vi "test_pid_1.vi"() -> ()   [LabVIEW 2018]
panel:
  out "Y":dbl[](graph)
  out "e(n)":dbl[](graph)
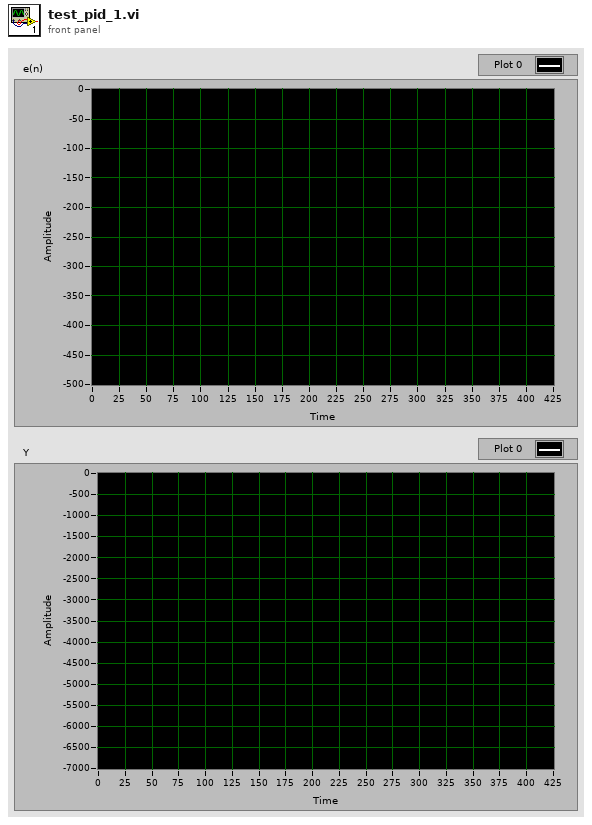
[diagram p1: front panel]
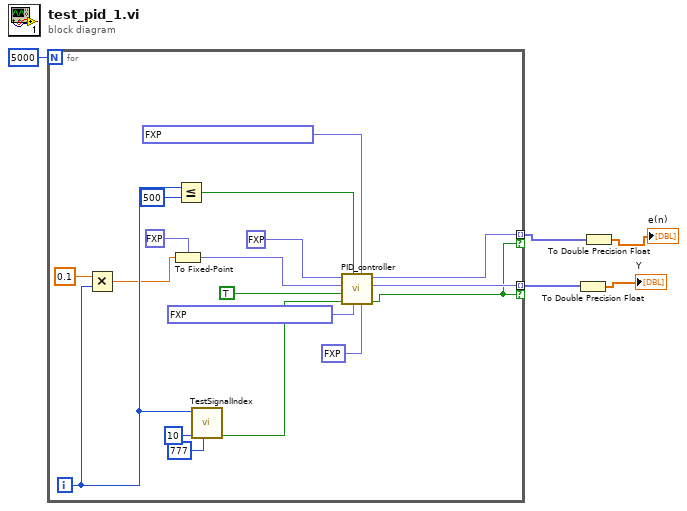
[diagram p0: block diagram]
diagram:
  n1 = for {
    N: 5000 -> [_]
    tunnel: [w9] -> w4 mode=indexing if=w7
    tunnel: [w8] -> w3 mode=indexing if=w7
    i -> [w16]
    n2 = Multiply(x=0.1, y=w16) -> (x*y=w13:dbl)
    n3 = To Fixed-Point(fixed-point type=fxp<+/-,32,14> 0.0 ("Y in"), number=w13) -> (fixed-point=w12:fxp<+/-,32,14>)
    n4 = Less Or Equal?(x=w16, y=500) -> (x <= y?=w19:bool)
    n5 = call "TestSignalIndex.vi"("initial delay"=777, "cycles per sample"=10, "index"=w16) -> ("valid out"=w21:bool)  [unwired: 7 in, 1 out]
    n6 = call "PID_controller.vi"("Kd/Tau"=fxp<+/-,32,13> 300.0, "Ki*Tau"=fxp<+/-,32,6> 0.01000000536441803, "Kp"=fxp<+/-,32,6> 0.09999999403953552, "Reset"=w19, "input valid"=w21, "Enabled"=TRUE, "Y in"=w12, "Ref in"=fxp<+/-,32,14> 0.0) -> ("output valid"=w7:bool, "Y out"=w8:fxp<+/-,32,14>, "e(n)"=w9:fxp<+/-,32,14>)  [unwired: 1 in]
  }
  n7 = To Double Precision Float(number=w3) -> (double precision float=→"Y":dbl[])
  n8 = To Double Precision Float(number=w4) -> (double precision float=→"e(n)":dbl[])
